vi "APC_Warning2DColorMap.vi"(1 "CylPresErrors":u64, 2 "CylPresWarnings":u64) -> (0 "Round Color Box":u32[][](array[colorbox]))   [LabVIEW 2020]
panel:
  out "Error":bool[][](array[boolean])
  out "Warning":bool[][](array[boolean])
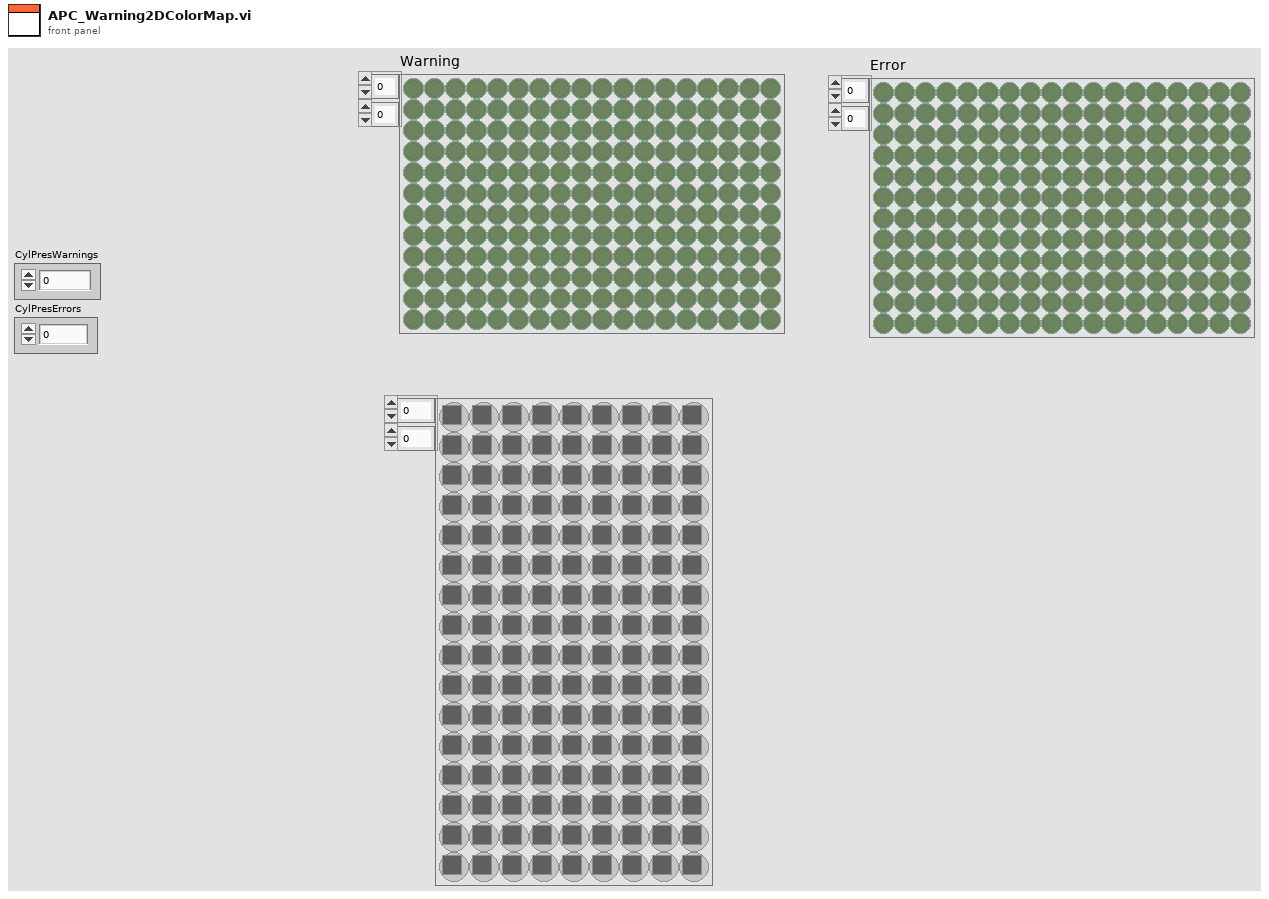
[diagram p1: front panel]
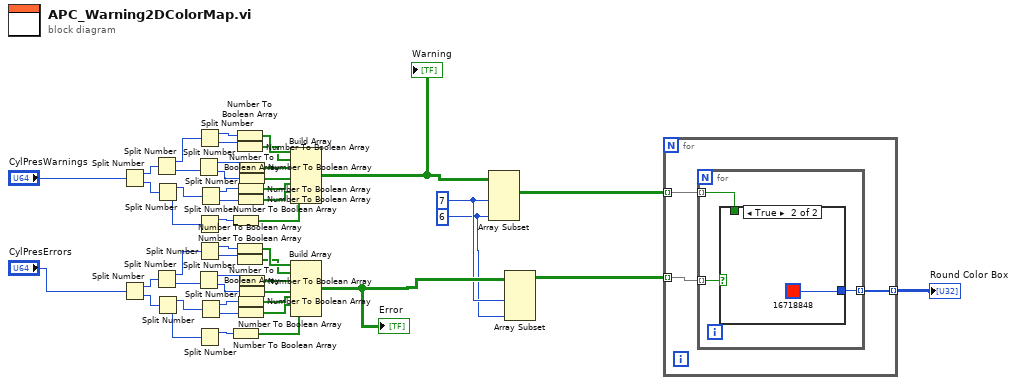
[diagram p0: block diagram]
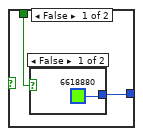
[diagram p2: hidden frame]
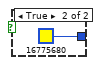
[diagram p3: hidden frame]
diagram:
  w1 = 6 ("length")
  w2 = 7 ("length")
  n1 = Split Number(x="CylPresWarnings") -> (hi(x)=w47:u32, lo(x)=w46:u32)
  n2 = Split Number(x="CylPresErrors") -> (hi(x)=w27:u32, lo(x)=w26:u32)
  n3 = Split Number(x=w47) -> (hi(x)=w45:u16, lo(x)=w44:u16)
  n4 = Split Number(x=w27) -> (hi(x)=w25:u16, lo(x)=w24:u16)
  n5 = Split Number(x=w46) -> (hi(x)=w43:u16, lo(x)=w42:u16)
  n6 = Split Number(x=w26) -> (hi(x)=w23:u16, lo(x)=w22:u16)
  n7 = Split Number(x=w44) -> (hi(x)=w39:u8, lo(x)=w38:u8)
  n8 = Split Number(x=w24) -> (hi(x)=w19:u8, lo(x)=w18:u8)
  n9 = Split Number(x=w45) -> (hi(x)=w41:u8, lo(x)=w40:u8)
  n10 = Split Number(x=w42) -> (hi(x)=w35:u8)  [unwired: 1 out]
  n11 = Split Number(x=w25) -> (hi(x)=w21:u8, lo(x)=w20:u8)
  n12 = Split Number(x=w22) -> (hi(x)=w15:u8)  [unwired: 1 out]
  n13 = Split Number(x=w43) -> (hi(x)=w37:u8, lo(x)=w36:u8)
  n14 = Split Number(x=w23) -> (hi(x)=w17:u8, lo(x)=w16:u8)
  n15 = Number To Boolean Array(number=w35) -> (Boolean array=w28:bool[])
  n16 = Number To Boolean Array(number=w15) -> (Boolean array=w8:bool[])
  n17 = Number To Boolean Array(number=w41) -> (Boolean array=w34:bool[])
  n18 = Number To Boolean Array(number=w40) -> (Boolean array=w33:bool[])
  n19 = Number To Boolean Array(number=w21) -> (Boolean array=w14:bool[])
  n20 = Number To Boolean Array(number=w20) -> (Boolean array=w13:bool[])
  n21 = Number To Boolean Array(number=w37) -> (Boolean array=w30:bool[])
  n22 = Number To Boolean Array(number=w36) -> (Boolean array=w29:bool[])
  n23 = Number To Boolean Array(number=w17) -> (Boolean array=w10:bool[])
  n24 = Number To Boolean Array(number=w16) -> (Boolean array=w9:bool[])
  n25 = Number To Boolean Array(number=w39) -> (Boolean array=w32:bool[])
  n26 = Number To Boolean Array(number=w38) -> (Boolean array=w31:bool[])
  n27 = Number To Boolean Array(number=w19) -> (Boolean array=w12:bool[])
  n28 = Number To Boolean Array(number=w18) -> (Boolean array=w11:bool[])
  n29 = Build Array(w34, w33, w32, w31, w30, w29, w28) -> (w6:bool[][])
  "Warning" <- w6
  n30 = Build Array(w14, w13, w12, w11, w10, w9, w8) -> (w3:bool[][])
  "Error" <- w3
  n31 = Array Subset(array=w6, length (row)=w2, length (col)=w1) -> (w5:bool[][])  [unwired: 2 in]
  n32 = Array Subset(array=w3, length (row)=w2, length (col)=w1) -> (w4:bool[][])  [unwired: 2 in]
  n33 = for {
    tunnel: w5 -> [w52] mode=indexing
    tunnel: w4 -> [w51] mode=indexing
    tunnel: [w50] -> w49 mode=indexing
    n34 = for {
      tunnel: w52 -> [w53] mode=indexing
      tunnel: w51 -> [w55] mode=indexing
      tunnel: [w54] -> w50 mode=indexing
      n35 = case shown="True" w55 {
        tunnel: [w56 u32 16718848 ("Round Color Box")] -> w54
        tunnel: w53 -> [w57 _]
        frame False {
          n36 = case shown="False" w57 {
            tunnel: [u32 6618880 ("Round Color Box") u32 16775680 ("Round Color Box")] -> w56
            frame False {
            }
            frame True {
            }
          }
        }
        frame True {
        }
      }
    }
  }
  "Round Color Box" <- w49
